vi "Measurement_PowerSupply.vi"(8 "error in (no error)":errorcluster {"code" format="%.0x"}, 9 "Channel_A":T1, 10 "Keysight PS":bool, 11 "VISA resource name":refnum<visa-resource-name>) -> (0 "error out":errorcluster {"code" format="%.0x"}, 1 "Current":dbl format="%^.3e", 2 "Voltage":dbl format="%^.3e", 3 "VISA resource name out":refnum<visa-resource-name>)   [LabVIEW 2018]
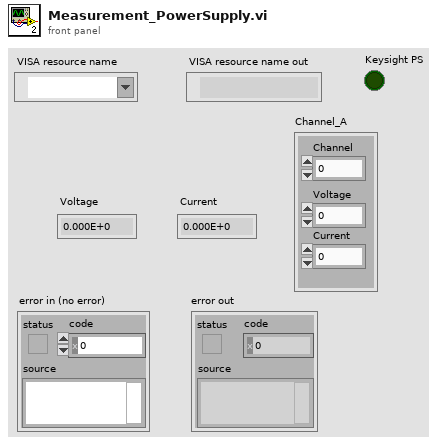
[diagram p1: front panel]
types:
  T1 = cluster{"Channel":dbl, "Voltage":dbl, "Current":dbl}
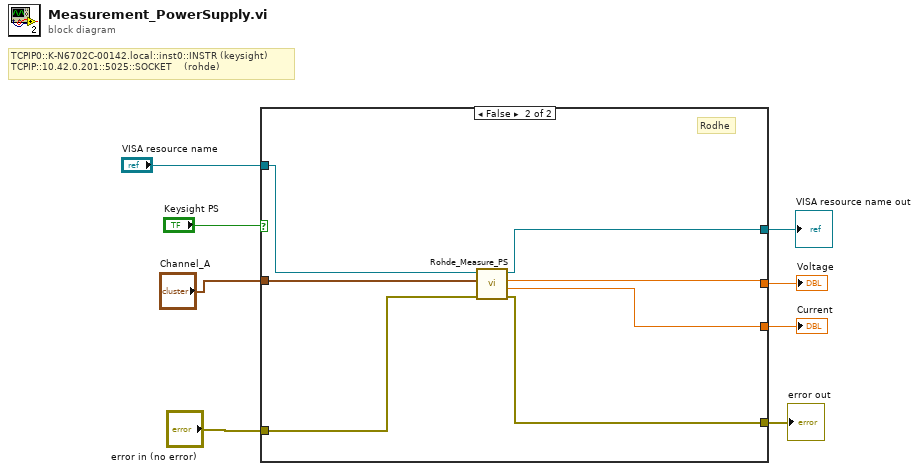
[diagram p0: block diagram]
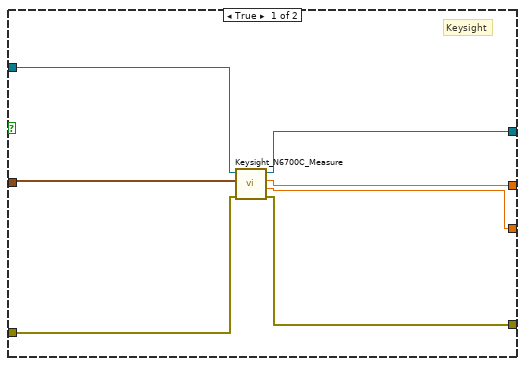
[diagram p2: hidden frame]
diagram:
  # "TCPIP0::K-N6702C-00142.local::inst0::INSTR (keysight)\nTCPIP::10.42.0.201::5025::SOCKET    (rohde)"
  n1 = case shown="False" "Keysight PS" {
    tunnel: "error in (no error)" -> [w15 w22]
    tunnel: [w11 w21] -> w7
    tunnel: [w14 w19] -> w5
    tunnel: [w13 w20] -> w4
    tunnel: [w12 w18] -> w3
    tunnel: "Channel_A" -> [w10 w17]
    tunnel: "VISA resource name" -> [w9 w16]
    frame True {
      # "Keysight"
      n2 = call "Keysight_N6700C_Measure.vi"("error in (no error)"=w15, "Channel_A"=w10, "VISA resource name"=w9) -> ("error out"=w14:errorcluster, "Current"=w12:dbl, "Voltage"=w13:dbl, "VISA resource name out"=w11:refnum<visa-resource-name>)  [unwired: 5 in]
    }
    frame False {
      # "Rodhe"
      n3 = call "Rohde_Measure_PS.vi"("error in (no error)"=w22, "Channel_A"=w17, "VISA resource name"=w16) -> ("error out"=w19:errorcluster, "Current (A)"=w18:dbl, "Voltage (V)"=w20:dbl, "PsAddressOut"=w21:refnum<visa-resource-name>)  [unwired: 4 in]
    }
  }
  "error out" <- w5
  "VISA resource name out" <- w7
  "Voltage" <- w4
  "Current" <- w3
